vi "test31-MappingRelationshipByLocalRegistration_WIthoutSubscriberName_State.vi"(8 "error in (no error)":errorcluster, 11 "TestCase in":refnum<class "testcase-CSMBroadcast.lvclass">) -> (0 "error out":errorcluster, 3 "TestCase out":refnum<class "testcase-CSMBroadcast.lvclass">)   [LabVIEW 2017, in "testcase-CSMBroadcast.lvclass"]
uses:
  testcase-CSMBroadcast.lvclass
  47fe1622-87c8-40c1-b9cf-9bbb5cd90bb5.vi
  <vilib>/addons/_JKI Toolkits/VI Tester/TestCase.llb/TestCase.lvclass
  src/user.lib/_NEVSTOP/Communicable State Machine(CSM)/Communicable State Machine.lvlib
  C:/Program Files (x86)/National Instruments/LabVIEW 2017/vi.lib/addons/_JKI Toolkits/VI Tester/TestCase.llb/TestCase.lvclass
  CSM/CSM-Testcase.lvlib
panel:
  out "Loop Count":i32
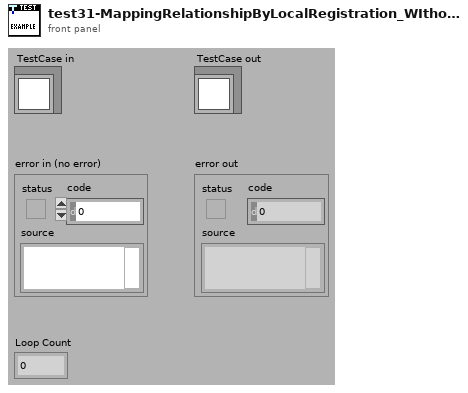
[diagram p1: front panel]
types:
  T1 = cluster{"Status":string, "Source CSM":string, "Target CSM":string, "Target API":string}[]
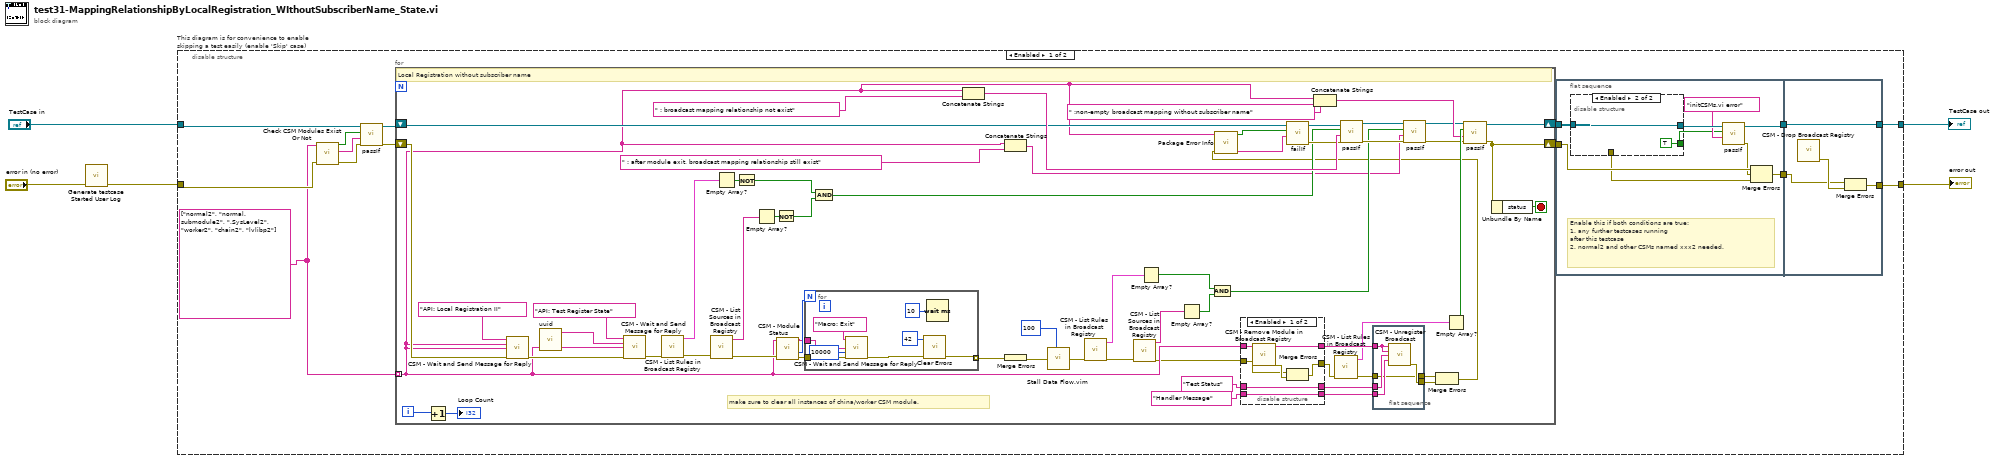
[diagram p0: block diagram]
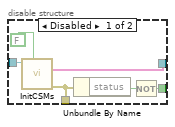
[diagram p2: hidden frame]
diagram:
  n1 = call "Generate testcase Started User Log.vi"("Error In"="error in (no error)") -> ("error out"=w1:errorcluster)  [unwired: 10 in]
  n2 = disable-structure "This diagram is for convenience to enable skipping a test easily (enable 'Skip' case)" shown="Enabled" {
    disable-tunnel: "TestCase in" -> [w16 w130]
    disable-tunnel: [w10 w128] -> w2
    disable-tunnel: [w9 w129] -> w4
    disable-tunnel: w1 -> [w15 w127]
    frame Enabled {
      w6 = string[] ["normal2", "normal.submodule2", ".SysLevel2", "worker2", "chain2", "lvlibp2"]
      n3 = call "Check CSM Modules Exist Or Not.vi"("error in"=w15, "CSM names in"=w6) -> ("error out"=w17:errorcluster, "Debug string"=w18:string, "All Modules Exist?"=w19:bool)  [unwired: 7 in]
      n4 = call-dynamic "passIf.vi"("error in (no error)"=w17, "message (\"\")"=w18, "pass"=w19, "TestCase in"=w16) -> ("error out"=w7:errorcluster, "TestCase out"=w8:refnum<class "testcase-CSMBroadcast.lvclass">)  [unwired: 6 in]
      n5 = for {
        tunnel: w6 -> [w46] mode=indexing
        shift-right: [w86] -> w12
        shift-left: w8 -> [w69]
        shift-right: [w87] -> w11
        shift-left: w7 -> [w84]
        i -> [w93]
        stop <- w96 stop-if-true
        # "make sure to clear all instances of china/worker CSM module."
        # "Local Registration without subscriber name"
        n6 = Increment(x=w93) -> (x+1=→"Loop Count":i32)
        n7 = call "CSM - Wait and Send Message for Reply.vi"("State"="API: Local Registration II", "Arguments (\"\")"=w46, "Target Module"=w46, "Error In (No Error)"=w84) -> ("error out"=w101:errorcluster)  [unwired: 8 in, 3 out]
        n8 = call "uuid.vi"() -> ("UUID"=w99:string)  [unwired: 11 in]
        n9 = call "CSM - Wait and Send Message for Reply.vi"("State"="API: Test Register State", "Arguments (\"\")"=w99, "Target Module"=w46, "Error In (No Error)"=w101) -> ("error out"=w98:errorcluster)  [unwired: 8 in, 3 out]
        n10 = call "CSM - List Rules in Broadcast Registry.vi"("error in (no error)"=w98) -> ("error out"=w95:errorcluster, "Rule Entries"=w91:T1)  [unwired: 8 in, 1 out]
        n11 = call "CSM - List Sources in Broadcast Registry.vi"("error in (no error)"=w95) -> ("error out"=w81:errorcluster, "Broadcast Names"=w88:string[])  [unwired: 9 in]
        n12 = Empty Array?(array=w91) -> (empty?=w90:bool)
        n13 = Not(x=w90) -> (.not. x?=w67:bool)
        n14 = Empty Array?(array=w88) -> (empty?=w89:bool)
        n15 = Not(x=w89) -> (.not. x?=w66:bool)
        n16 = call "CSM - Module Status.vi"("Error In"=w81, "CSM Name"=w46) -> ("error out"=w80:errorcluster, "#Nodes"=w83:i32, "CSM Name (Dup)"=w82:string)  [unwired: 5 in, 2 out]
        n17 = for {
          N: w83 -> [_]
          tunnel: [w121] -> w97 mode=indexing
          tunnel: w82 -> [w125]
          tunnel: w80 -> [w124]
          n18 = call "CSM - Wait and Send Message for Reply.vi"("State"="Macro: Exit", "Target Module"=w125, "Wait (5000ms)"=10000, "Error In (No Error)"=w124) -> ("error out"=w122:errorcluster)  [unwired: 8 in, 3 out]
          n19 = call <vilib>:"Clear Errors.vi"("error in (no error)"=w122, "specific error code to clear (0: all)"=42) -> ("error out"=w121:errorcluster)  [unwired: 4 in, 1 out]
          n20 = Wait (ms)(milliseconds to wait=u32 10) -> ()  [unwired: 1 out]
        }
        n21 = And(x=w67, y=w66) -> (x .and. y?=w65:bool)
        n22 = Concatenate Strings(w46, " : broadcast mapping relationship not exist" ("string")) -> (w76:string)
        n23 = Concatenate Strings(w46, " : after module exit, broadcast mapping relationship still exist" ("string")) -> (w54:string)
        n24 = Merge Errors(w97) -> (w75:errorcluster)
        n25 = call "Stall Data Flow.vim"("value in"=w75, "milliseconds to wait"=u32 100) -> ("value out"=w74:errorcluster)  [unwired: 1 out]
        n26 = call "CSM - List Rules in Broadcast Registry.vi"("error in (no error)"=w74) -> ("error out"=w94:errorcluster, "Rule Entries"=w60:T1)  [unwired: 8 in, 1 out]
        n27 = call "CSM - List Sources in Broadcast Registry.vi"("error in (no error)"=w94) -> ("error out"=w45:errorcluster, "Broadcast Names"=w59:string[])  [unwired: 9 in]
        n28 = Empty Array?(array=w60) -> (empty?=w58:bool)
        n29 = Empty Array?(array=w59) -> (empty?=w57:bool)
        n30 = And(x=w58, y=w57) -> (x .and. y?=w56:bool)
        n31 = disable-structure shown="Enabled" {
          disable-tunnel: w45 -> [w108 w117]
          disable-tunnel: [w112 w117] -> w52
          disable-tunnel: w46 -> [w113 w118]
          disable-tunnel: "Test Status" ("Status") -> [w110 w116]
          disable-tunnel: "Handler Message" ("Response Message (If \"\", Same as Source Message)") -> [w109 w115]
          disable-tunnel: [w111 w118] -> w53
          disable-tunnel: [w110 w116] -> w51
          disable-tunnel: [w109 w115] -> w50
          frame Enabled {
            n32 = call "CSM - Remove Module in Broadcast Registry.vi"("CSM Name"=w113) -> ("CSM Name (Dup)"=w111:string, "error out"=w114:errorcluster)  [unwired: 13 in]
            n33 = Merge Errors(w108, w114) -> (w112:errorcluster)
          }
          frame Disabled {
          }
        }
        n34 = Concatenate Strings(w46, " :non-empty broadcast mapping without subscriber name" ("string")) -> (w77:string)
        n35 = call "CSM - List Rules in Broadcast Registry.vi"("error in (no error)"=w52) -> ("error out"=w48:errorcluster, "Rule Entries"=w41:T1)  [unwired: 8 in, 1 out]
        n36 = flat-sequence {
          tunnel: w53 -> [w107]
          tunnel: w51 -> [w106]
          tunnel: w50 -> [w105]
          tunnel: [w104] -> w49
          tunnel: w48 -> [w103]
          tunnel: [w103] -> w47
          frame #0 {
            n37 = call "CSM - Unregister Broadcast.vi"("CSM Name(Empty for Broadcast Event)"=w107, "Source CSM Name (* as Default)"=w107, "Trigger"=w106, "API (\"*\" as Default)"=w105) -> ("error out"=w104:errorcluster)  [unwired: 10 in, 1 out]
          }
        }
        n38 = Merge Errors(w47, w49) -> (w44:errorcluster)
        n39 = call "Package Error Info.vi"("error in"=w44, "String in"=w46) -> ("packed error info out"=w72:string, "error status"=w71:bool)  [unwired: 8 in]
        n40 = call-dynamic "failIf.vi"("message (\"\")"=w72, "fail"=w71, "TestCase in"=w69) -> ("error out"=w70:errorcluster, "TestCase out"=w68:refnum<class "testcase-CSMBroadcast.lvclass">)  [unwired: 7 in]
        n41 = call-dynamic "passIf.vi"("error in (no error)"=w70, "message (\"\")"=w76, "pass"=w65, "TestCase in"=w68) -> ("error out"=w62:errorcluster, "TestCase out"=w64:refnum<class "testcase-CSMBroadcast.lvclass">)  [unwired: 6 in]
        n42 = call-dynamic "passIf.vi"("error in (no error)"=w62, "message (\"\")"=w54, "pass"=w56, "TestCase in"=w64) -> ("error out"=w61:errorcluster, "TestCase out"=w63:refnum<class "testcase-CSMBroadcast.lvclass">)  [unwired: 6 in]
        n43 = Empty Array?(array=w41) -> (empty?=w85:bool)
        n44 = call-dynamic "passIf.vi"("error in (no error)"=w61, "message (\"\")"=w77, "pass"=w85, "TestCase in"=w63) -> ("error out"=w87:errorcluster, "TestCase out"=w86:refnum<class "testcase-CSMBroadcast.lvclass">)  [unwired: 6 in]
        n45 = Unbundle By Name(w87) -> ("status"=w96:bool)
      }
      n46 = flat-sequence {
        tunnel: w12 -> [w28]
        tunnel: [w26] -> w14
        tunnel: w11 -> [w24]
        tunnel: [w21] -> w13
        tunnel: w14 -> [w39]
        tunnel: [w39] -> w10
        tunnel: [w38] -> w9
        tunnel: w13 -> [w37]
        frame #0 {
          # "Enable this if both conditions are true:\n1. any further testcases running\nafter this testcase\n2. normal2 and other CSMs named xxx2 needed."
          n47 = disable-structure shown="Enabled" {
            disable-tunnel: w28 -> [w34 w36]
            disable-tunnel: [w32 w36] -> w27
            disable-tunnel: [w30 _] -> w22
            disable-tunnel: [w29 TRUE ("pass")] -> w20
            frame Disabled {
              n48 = call "InitCSMs.vi"(7:FALSE ("Enable building lvlibp?"), 11:w34) -> ("error out"=w30:errorcluster, "CSMs"=w32:string[])  [unwired: 8 in]
              n49 = Unbundle By Name(w30) -> ("status"=w31:bool)
              n50 = Not(x=w31) -> (.not. x?=w29:bool)
            }
            frame Enabled {
            }
          }
          n51 = call-dynamic "passIf.vi"("message (\"\")"="initCSMs.vi error" ("message (\"\")"), "pass"=w20, "TestCase in"=w27) -> ("error out"=w23:errorcluster, "TestCase out"=w26:refnum<class "testcase-CSMBroadcast.lvclass">)  [unwired: 7 in]
          n52 = Merge Errors(w24, w23, w22) -> (w21:errorcluster)
        }
        frame #1 {
          n53 = call "CSM - Drop Broadcast Registry.vi"() -> ("error out"=w40:errorcluster)  [unwired: 15 in]
          n54 = Merge Errors(w37, w40) -> (w38:errorcluster)
        }
      }
    }
    frame Disabled {
      # "skip test result while test is under development"
      n55 = call <vilib>:"skip.vi"("error in (no error)"=w127, "TestCase in"=w130) -> ("error out"=w129:errorcluster, "TestCase out"=w128:refnum<class "testcase-CSMBroadcast.lvclass">)  [unwired: 8 in]
    }
  }
  "error out" <- w4
  "TestCase out" <- w2
